vi "example1.vi"() -> ()   [LabVIEW 2024]
panel:
  in  "Array":dbl[](array[numeric])
  out "Waveform Graph":dbl[](graph)
  out "Waveform Chart":dbl(graph)
  # "In this  Vi, I implemented the logic\n to clear the history \neverytime before the\n loop runs."
  # "In this VI,  sin values are generated and connected a waveform chart and waveform graph for the values\n1. Using the data in the graph we can export the values into excel or into images or u can save to clip board.\nright click on the graph->export option->and you can see multile  options."
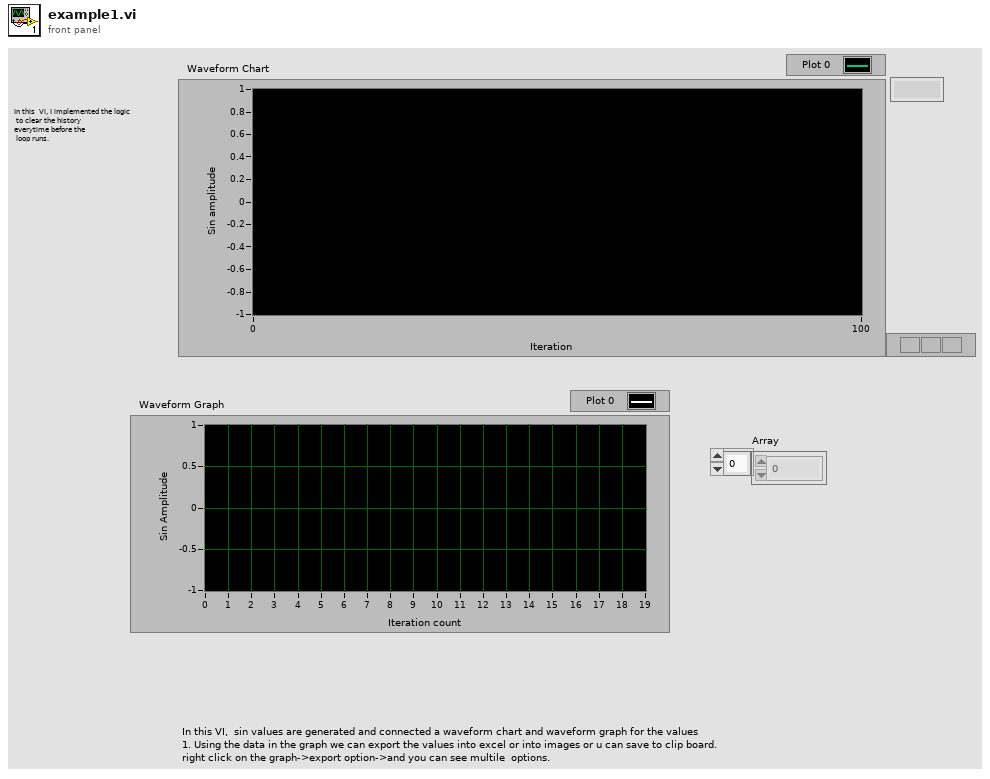
[diagram p1: front panel]
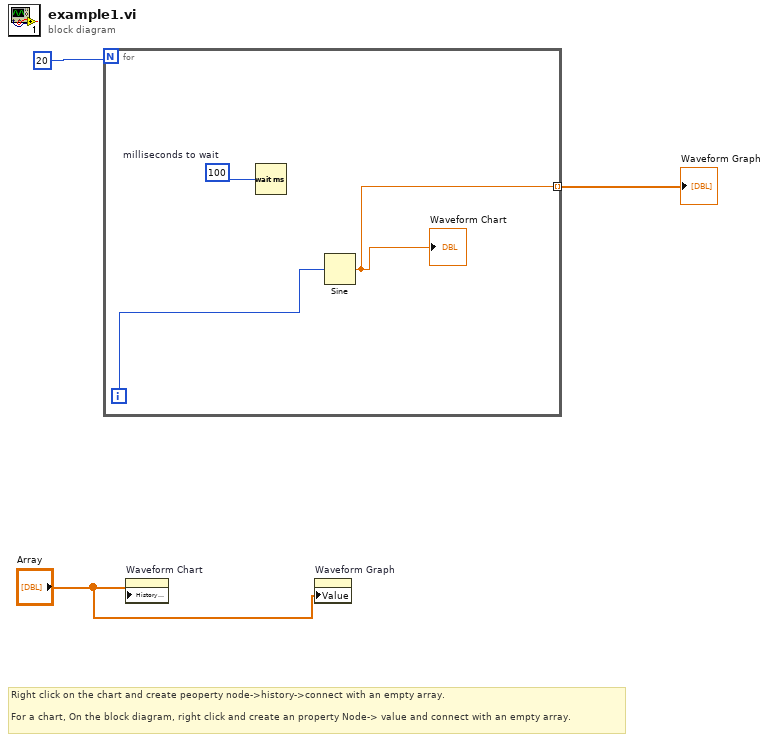
[diagram p0: block diagram]
diagram:
  # "Right click on the chart and create peoperty node->history->connect with an empty array.\n\nFor a chart, On the block diagram, right click and create an property Node-> value and connect with an empty array."
  n1 = for {
    N: 20 -> [_]
    tunnel: [w4] -> w2 mode=indexing
    i -> [w5]
    w6 = u32 100  # milliseconds to wait
    n2 = Wait (ms)(milliseconds to wait=w6) -> ()  [unwired: 1 out]
    n3 = Sine(x=w5) -> (sin(x)=w4:dbl)
    "Waveform Chart" <- w4
  }
  "Waveform Graph" <- w2
  n4 = property on="Waveform Chart" class="WFChart (strict)"("History Data"="Array") -> ()  [unwired: 2 in, 2 out]
  n5 = property on="Waveform Graph" class="WFGraph (strict)"("Value"="Array") -> ()  [unwired: 2 in, 2 out]
